vi "Read channel info.vi"(8 "error in (no error)":errorcluster, 11 "DSFChannel in":refnum<class "DSFChannel.lvclass">) -> (0 "error out":errorcluster, 2 "channel info":T1, 3 "DSFChannel out":refnum<class "DSFChannel.lvclass">)   [LabVIEW 2017, in "DSFChannel.lvclass"]
uses:
  DSFChannel.lvclass
  Controls/dsf configuration file/1.0.0/dsf channel.ctl
  DSFChannel.lvclass/DSFChannel.ctl
  Controls/dsf configuration file/1.0.0/dsf configuration file v1.0.0.lvlib
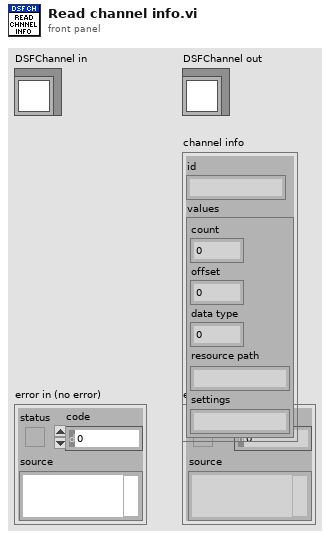
[diagram p1: front panel]
types:
  T1 = typedef "dsf configuration file v1.0.0.lvlib/dsf channel.ctl" = cluster{"id":string, "values":cluster{"count":i32, "offset":i32, "data type":dbl, "resource path":string, "settings":string}}
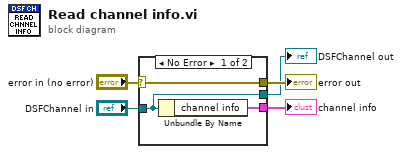
[diagram p0: block diagram]
diagram:
  n1 = case shown="No Error" "error in (no error)" {
    selector: "error in (no error)" -> [w8 w9]
    tunnel: [w8 w9] -> w4
    tunnel: [w7 w10] -> w2
    tunnel: "DSFChannel in" -> [w7 w10]
    tunnel: [w6 _] -> w1
    frame No Error {
      n2 = Unbundle By Name(w7) -> ("channel info"=w6:T1)
    }
    frame Error {
    }
  }
  "error out" <- w4
  "DSFChannel out" <- w2
  "channel info" <- w1
